vi "Load Config.vi"(8 "error in (no error)":errorcluster, 11 "Telemetry Server Module in":refnum<class "Telemetry Server Module.lvclass">) -> (0 "error out":errorcluster, 3 "Telemetry Server Module out":refnum<class "Telemetry Server Module.lvclass">)   [LabVIEW 2020, in "Volatus.lvlib" / "Telemetry Server Module.lvclass"]
uses:
  Telemetry Server Module.lvclass
  C:/dev/lv20CE/relink/lv-volatus/Volatus/Module/Module.lvclass
  VolatusConfig/Meta Type.ctl
  Module/Module.lvclass/Module.ctl
  VolatusConfig/VolatusConfigElement/VolatusConfigElement.lvclass/VolatusConfigElement.ctl
  Telemetry Server Module.lvclass/Telemetry Server Module.ctl
  Module/Config.vi
  VolatusConfig/VolatusConfigElement/Element.vi
  VolatusConfig/Task/Task Config.lvclass
  C:/dev/lv20CE/relink/lv-volatus/VolatusConfig/VolatusConfigElement/VolatusConfigElement.lvclass
  lv-cdm/CDM-Config/Config Lookup/Match Meta.vi
  lv-cdm/CDM-Config/Config Element/Owner.vi
  lv-cdm/CDM-Config/Config Filter/Config Lookup.lvclass
  Module/Module.lvclass
  VolatusConfig/VolatusConfigElement/VolatusConfigElement.lvclass
  VolatusConfig/VolatusConfig.lvlib
  VolatusConfig/Cluster/Cluster Config.lvclass
  lv-vecto/Vecto/IP Resolver/IP Resolver.lvclass
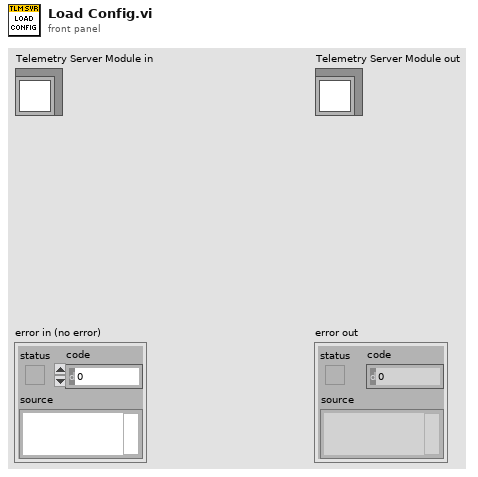
[diagram p1: front panel]
types:
  T1 = typedef "VolatusConfig.lvlib/Meta Type.ctl" = enum16{"UNKNOWN", "VL_System", "VL_Cluster", "VL_Node", "VL_Task", "VL_Group", "VL_Channel", "VL_Task_List", "VL_Scaling", "VL_Sensor", "VL_Sensor_List", "VL_Scale"}
  T2 = typedef "VectoConfig.lvlib/Telemetry Config.ctl" = cluster{"Routing":T3, "Endpoint":T4}
  T3 = typedef "VectoConfig.lvlib/Telemetry Routing.ctl" = enum16{"Multicast", "Unicast"}
  T4 = typedef "VectoConfig.lvlib/Endpoint.ctl" = cluster{"Address":string, "Port":u16}
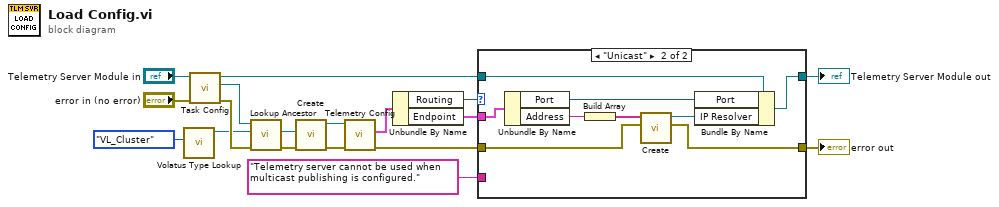
[diagram p0: block diagram]
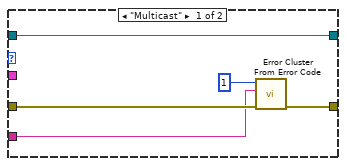
[diagram p2: hidden frame]
diagram:
  n1 = call "Volatus Type Lookup.vi"("Meta Type"=Meta_Type."VL_Cluster") -> ("Config Lookup out"=w14:refnum<class "Config Lookup.lvclass">)  [unwired: 9 in, 1 out]
  n2 = call "Task Config.vi"("error in (no error)"="error in (no error)", "Module in"="Telemetry Server Module in") -> ("error out"=w18:errorcluster, "Task Config"=w15:refnum<class "Task Config.lvclass">, "Module out"=w5:refnum<class "Telemetry Server Module.lvclass">)  [unwired: 7 in]
  n3 = call "Lookup Ancestor.vi"("error in (no error)"=w18, "Lookup"=w14, "VolatusConfigElement in"=w15) -> ("error out"=w11:errorcluster, "Ancestor"=w12:refnum<class "Config Element.lvclass">)  [unwired: 6 in, 1 out]
  n4 = call "Create.vi"("error in (no error)"=w11, "Element"=w12) -> ("error out"=w10:errorcluster, "Cluster out"=w9:refnum<class "Cluster Config.lvclass">)  [unwired: 8 in]
  n5 = call "Telemetry Config.vi"("error in (no error)"=w10, "Cluster Config in"=w9) -> ("error out"=w4:errorcluster, "Telemetry Config"=w8:T2)  [unwired: 7 in, 1 out]
  n6 = Unbundle By Name(w8) -> ("Routing"=w7:T3, "Endpoint"=w6:T4)
  n7 = case shown="\"Unicast\"" w7 {
    tunnel: w6 -> [_ w30]
    tunnel: w5 -> [w23 w32]
    tunnel: w4 -> [w22 w25]
    tunnel: [w23 w31] -> w3
    tunnel: [w20 w24] -> w2
    tunnel: "Telemetry server cannot be used when multicast publishing is configured." -> [w19 _]
    frame "Multicast" {
      n8 = call <vilib>:"Error Cluster From Error Code.vi"("error in (no error)"=w22, "error message (\"\")"=w19, "error code (0)"=1) -> ("error out"=w20:errorcluster)  [unwired: 6 in]
    }
    frame "Unicast" {
      n9 = Unbundle By Name(w30) -> ("Port"=w29:u16, "Address"=w28:string)
      n10 = Build Array(w28) -> (w26:string[])
      n11 = call "Create.vi"("error in (no error)"=w25, "Bindings"=w26) -> ("error out"=w24:errorcluster, "IP Resolver"=w27:refnum<class "IP Resolver.lvclass">)  [unwired: 8 in]
      n12 = Bundle By Name(cluster=w32, "Port"=w29, "IP Resolver"=w27) -> (w31:refnum<class "Telemetry Server Module.lvclass">)
    }
  }
  "error out" <- w2
  "Telemetry Server Module out" <- w3
